vi "Import.vi"(8 "error in":errorcluster, 11 "Objects":T1) -> (0 "error out":errorcluster, 1 "Success?":bool)   [LabVIEW 2017, in "J1939 editor node.lvclass"]
uses:
  J1939 editor node.lvclass
  <vilib>/NI/DCAF/Tag Editor Core/Table API/Table Manager/object ref.ctl
  <vilib>/NI/DCAF/Tag Editor Core/Configuration Editor/Classes/Engine Parent/Engine Parent Editor Node.lvclass
  <vilib>/NI/DCAF/Tag Editor Core/Configuration Editor/Classes/Module editor node/module editor node.lvclass
  <vilib>/NI/DCAF/Tag Editor Core/Table API/Table Manager/Table Manager.lvclass
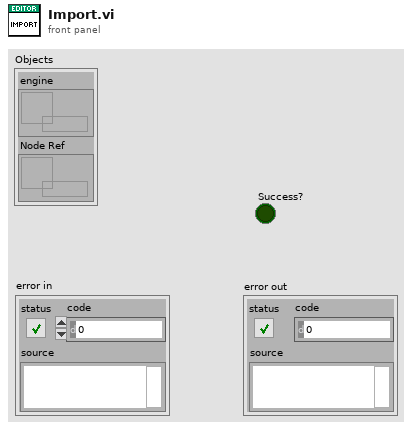
[diagram p1: front panel]
types:
  T1 = typedef "Table Manager.lvlib/Table Manager.lvclass/object ref.ctl" = cluster{"engine":refnum<data-value>, "Node Ref":refnum<data-value>}
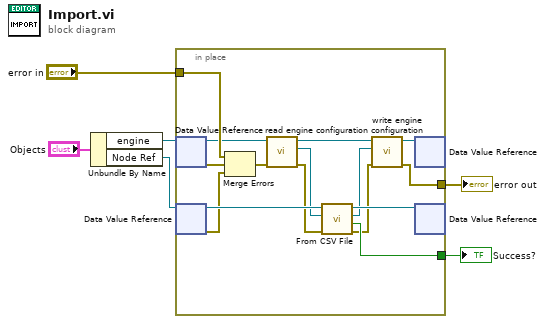
[diagram p0: block diagram]
diagram:
  n1 = Unbundle By Name("Objects") -> ("engine"=w5:refnum<data-value>, "Node Ref"=w1:refnum<data-value>)
  n2 = in-place {
    in-place-border: [w10] -> w4
    in-place-border: "error in" -> [w19]
    in-place-border: [w18] -> w2
    n3 = in-place-dvr #1(w5) -> (w17:refnum<class "Engine Parent Editor Node.lvclass">, w8:errorcluster)
    n4 = in-place-dvr #2(w1) -> (w21:refnum<class "module editor node.lvclass">, w7:errorcluster)
    n5 = Merge Errors(w19, w8, w7) -> (w14:errorcluster)
    n6 = call <vilib>:"read engine configuration.vi"("error in"=w14, "Engine Parent Editor Node in"=w17) -> ("error out"=w15:errorcluster, "engine configuration"=w16:refnum<class "engine configuration.lvclass">, "Engine Parent Editor Node out"=w13:refnum<class "Engine Parent Editor Node.lvclass">)  [unwired: 7 in]
    n7 = call-dynamic "From CSV File.vi"("error in (no error)"=w15, "engine in"=w16, "module editor node in"=w21) -> ("error out"=w11:errorcluster, "Update"=w18:bool, "engine out"=w12:refnum<class "engine configuration.lvclass">, "module editor node out"=w20:refnum<class "module editor node.lvclass">)  [unwired: 5 in]
    n8 = call <vilib>:"write engine configuration.vi"("error in"=w11, "engine configuration"=w12, "Engine Parent Editor Node in"=w13) -> ("error out"=w10:errorcluster, "Engine Parent Editor Node out"=w9:refnum<class "Engine Parent Editor Node.lvclass">)  [unwired: 7 in]
    n9 = in-place-dvr #1(w9) -> ()  [unwired: 2 out]
    n10 = in-place-dvr #2(w20) -> ()  [unwired: 2 out]
  }
  "Success?" <- w2
  "error out" <- w4
